vi "Power Brake.vi"(1 "Arm Speed":dbl) -> (0 "Final Speed Value":dbl)   [LabVIEW 2018]
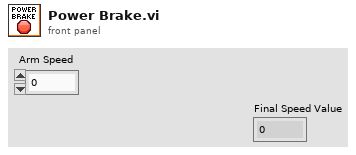
[diagram p1: front panel]
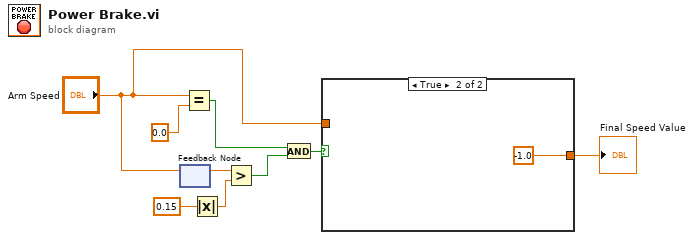
[diagram p0: block diagram]
diagram:
  n1 = feedback #1() -> (w6:dbl)  [unwired: 1 in]
  n2 = feedback-in #1("Arm Speed") -> ()
  n3 = Equal?(x="Arm Speed", y=0.0) -> (x = y?=w8:bool)
  n4 = Absolute Value(x=0.15) -> (abs(x)=w5:dbl)
  n5 = Greater?(x=w6, y=w5) -> (0:w7:bool)
  n6 = And(x=w8, y=w7) -> (x .and. y?=w3:bool)
  n7 = case shown="True" w3 {
    tunnel: [w10 -1.0] -> w2
    tunnel: "Arm Speed" -> [w10 _]
    frame False {
    }
    frame True {
    }
  }
  "Final Speed Value" <- w2
